vi "HeaterConfigurationGlobal.vi"(6 "Index":i32, 7 "Action":T2=enum."Get", 11 "Set Value":T1={"COM Port"=1, "Setpoint"=0.0, "Standby?"=FALSE}) -> (3 "Value Out":T1={"COM Port"=1, "Setpoint"=0.0, "Standby?"=FALSE})   [LabVIEW 2012]
uses:
  HeaterConfigurationGlobalAction.ctl
  HeaterConfiguration.ctl
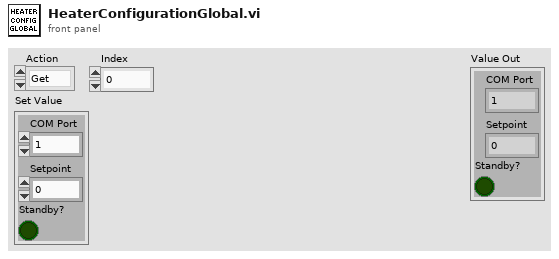
[diagram p1: front panel]
types:
  T1 = typedef "HeaterConfiguration.ctl" = cluster{"COM Port":u8, "Setpoint":dbl, "Standby?":bool}
  T2 = typedef "HeaterConfigurationGlobalAction.ctl" = enum16{"Init", "Get", "Set", "Add", "Remove", "Reset"}
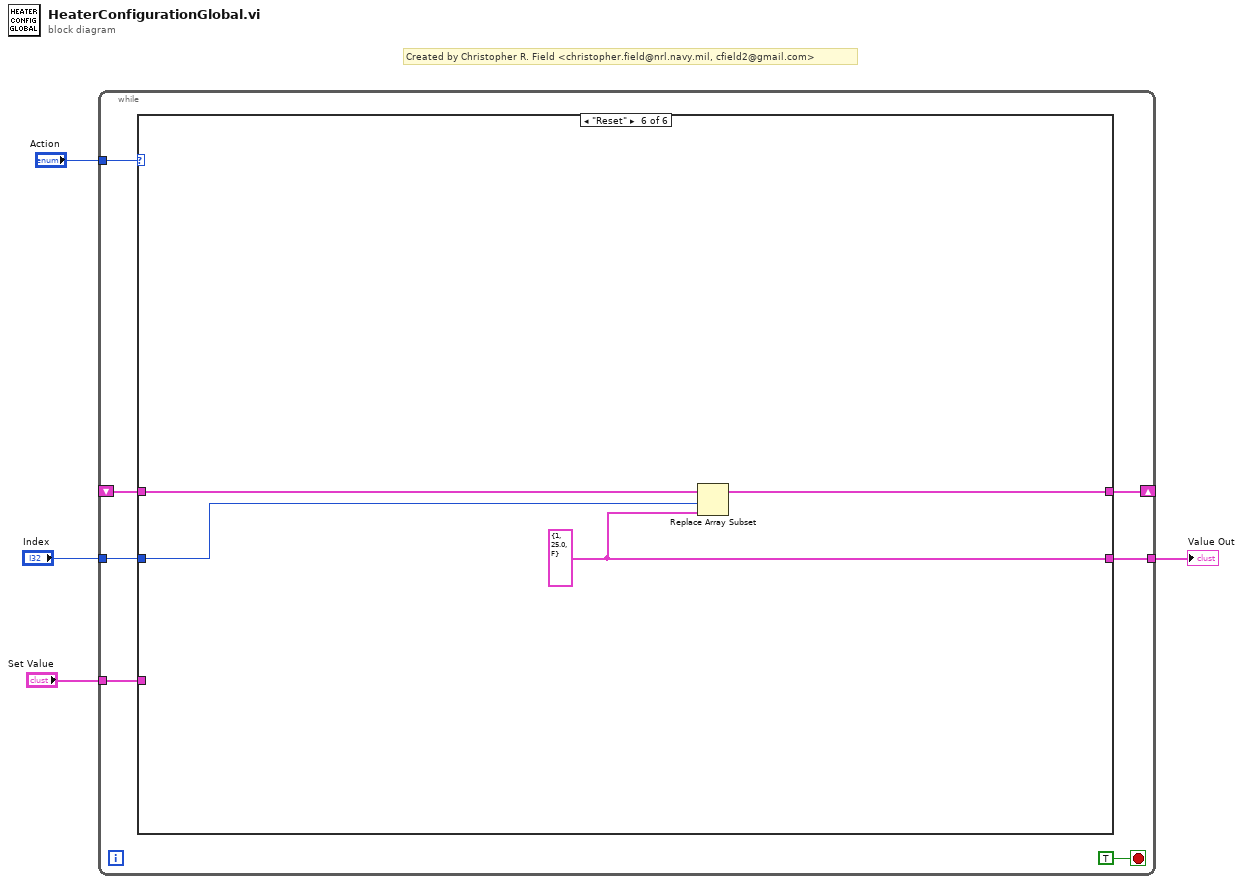
[diagram p0: block diagram]
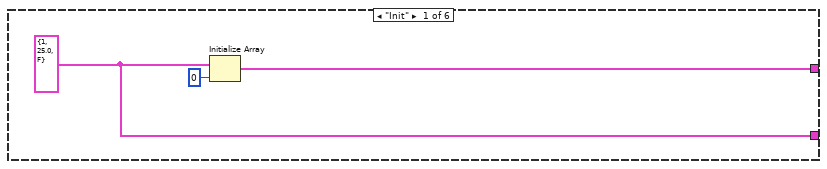
[diagram p2: hidden frame]
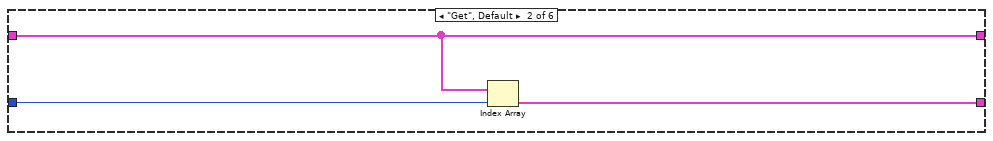
[diagram p3: hidden frame]
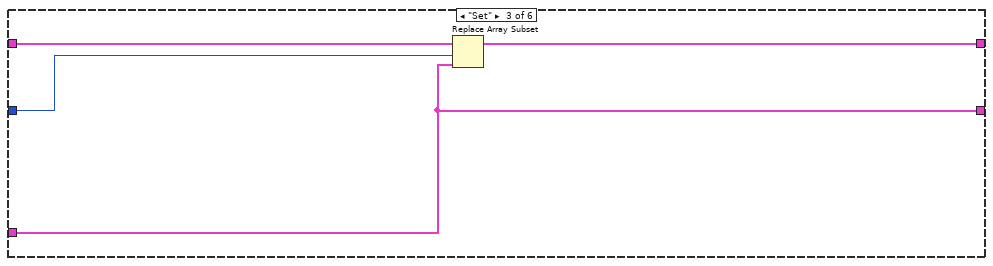
[diagram p4: hidden frame]
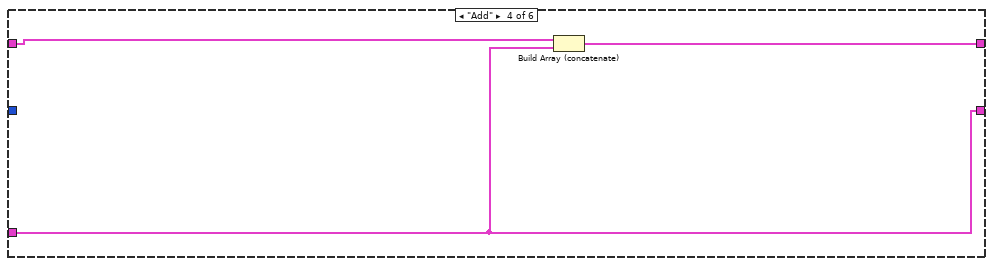
[diagram p5: hidden frame]
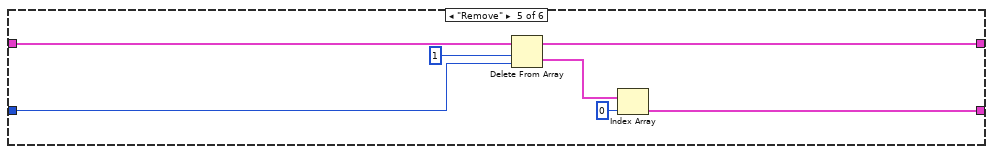
[diagram p6: hidden frame]
diagram:
  # "Created by Christopher R. Field <christopher.field@nrl.navy.mil, cfield2@gmail.com>"
  n1 = while {
    tunnel: "Action" -> [w10]
    tunnel: "Set Value" -> [w9]
    shift-right: [w8] -> _
    shift-left: _ -> [w7]
    tunnel: "Index" -> [w6]
    tunnel: [w5] -> w1
    stop <- TRUE stop-if-true
    n2 = case shown="\"Reset\"" w10 {
      tunnel: w9 -> [_ _ w18 w22 _ _]
      tunnel: [w13 w17 w20 w24 w28 w33] -> w8
      tunnel: w7 -> [_ w17 w21 w23 w31 w35]
      tunnel: w6 -> [_ w16 w19 _ w29 w34]
      tunnel: [w12 w15 w18 w22 w25 w32] -> w5
      frame "Init" {
        w12 = T1 {"COM Port"=1, "Setpoint"=25.0, "Standby?"=FALSE} ("Set Value")
        n3 = Initialize Array(w12, 0 ("dimension size")) -> (w13:T1[])
      }
      frame "Get", Default {
        n4 = Index Array(array=w17, index=w16) -> (element=w15:T1)
      }
      frame "Set" {
        n5 = Replace Array Subset(array=w21, new element=w18, index=w19) -> (w20:T1[])
      }
      frame "Add" {
        n6 = Build Array (concatenate)(w23, w22) -> (w24:T1[])
      }
      frame "Remove" {
        n7 = Delete From Array(array=w31, length=1, index=w29) -> (deleted portion=w27:T1[], array with subset deleted=w28:T1[])
        n8 = Index Array(array=w27, index=0) -> (element=w25:T1)
      }
      frame "Reset" {
        w32 = T1 {"COM Port"=1, "Setpoint"=25.0, "Standby?"=FALSE} ("Set Value")
        n9 = Replace Array Subset(array=w35, new element=w32, index=w34) -> (w33:T1[])
      }
    }
  }
  "Value Out" <- w1
